vi "onCheckConnection.vi"(8 "error in (no error)":errorcluster, 11 "Connection.LocalQueue":refnum<class "Connection.NetworkStream.lvclass">) -> (0 "error out":errorcluster, 1 "Outbound connection OK":bool, 2 "Inbound connection OK":bool, 3 "Connection.LocalQueue":refnum<class "Connection.NetworkStream.lvclass">)   [LabVIEW 2013, in "Connection.NetworkQueue_GOSPL.lvlib" / "Connection.NetworkStream.lvclass"]
uses:
  Connection.NetworkStream/Connection.NetworkStream.lvclass
  Connection.NetworkStream/Connection.NetworkStream.lvclass/Connection.NetworkStream.ctl
  <resource>/objmgr/ni.dex.rc
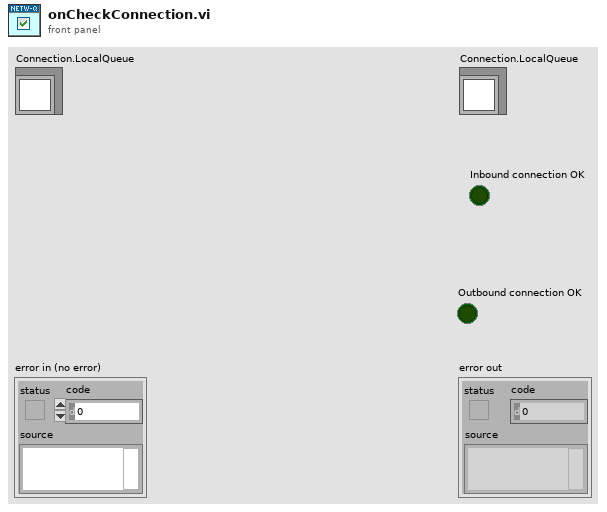
[diagram p1: front panel]
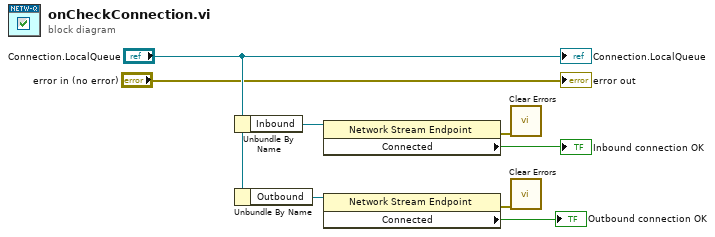
[diagram p0: block diagram]
diagram:
  n1 = Unbundle By Name("Connection.LocalQueue") -> ("Inbound"=w5:refnum<k21>)
  n2 = Unbundle By Name("Connection.LocalQueue") -> ("Outbound"=w4:refnum<k21>)
  n3 = property class="Network Stream Endpoint"(reference=w5) -> (error out=w2:errorcluster, "Connected"=→"Inbound connection OK":bool)  [unwired: 1 in, 1 out]
  n4 = property class="Network Stream Endpoint"(reference=w4) -> (error out=w1:errorcluster, "Connected"=→"Outbound connection OK":bool)  [unwired: 1 in, 1 out]
  n5 = call <vilib>:"Clear Errors.vi"("error in (no error)"=w2) -> ()  [unwired: 6 in, 1 out]
  n6 = call <vilib>:"Clear Errors.vi"("error in (no error)"=w1) -> ()  [unwired: 6 in, 1 out]
  "error out" <- "error in (no error)"
  "Connection.LocalQueue" <- "Connection.LocalQueue"
